vi "setBuffer.vi"(10 "Buffer":u16[](array[numeric]), 11 "ModbusBuffer in":refnum<class "ModbusBuffer.lvclass">) -> (3 "ModbusBuffer out":refnum<class "ModbusBuffer.lvclass">)   [LabVIEW 2016, in "RTModbus.lvlib" / "ModbusBuffer.lvclass"]
uses:
  ModbusBuffer.lvclass
  ModbusBuffer.lvclass/ModbusBuffer.ctl
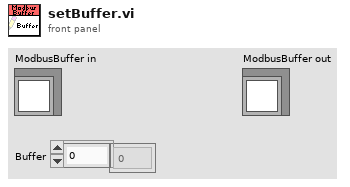
[diagram p1: front panel]
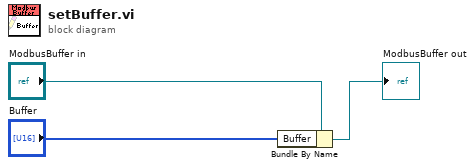
[diagram p0: block diagram]
diagram:
  n1 = Bundle By Name(cluster="ModbusBuffer in", "Buffer"="Buffer") -> (→"ModbusBuffer out":refnum<class "ModbusBuffer.lvclass">)
